vi "amp e offset control.vi"(8 "amp ref":refnum<vi>, 9 "Amplitude (Vp)":dbl, 10 "Offset (V)":dbl, 11 "offset ref":refnum<vi>) -> (1 "Nova Amplitude":dbl, 2 "Novo Offset":dbl)   [LabVIEW 2019]
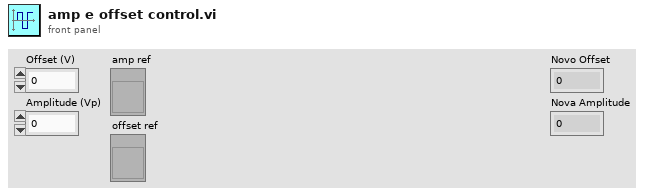
[diagram p1: front panel]
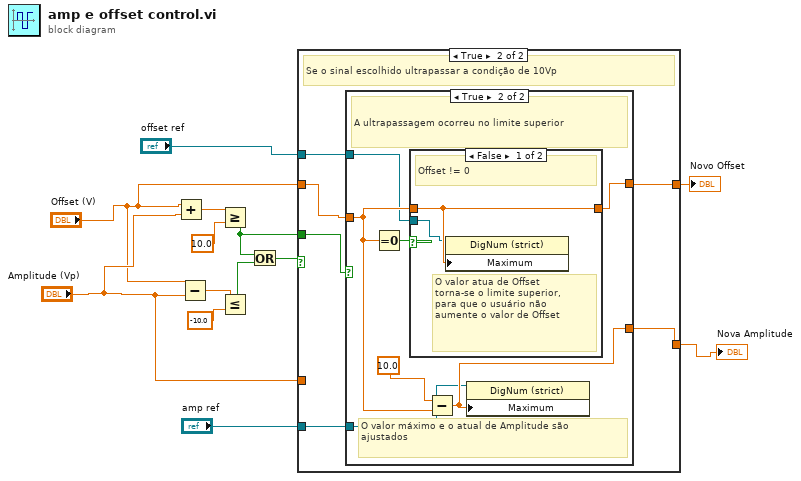
[diagram p0: block diagram]
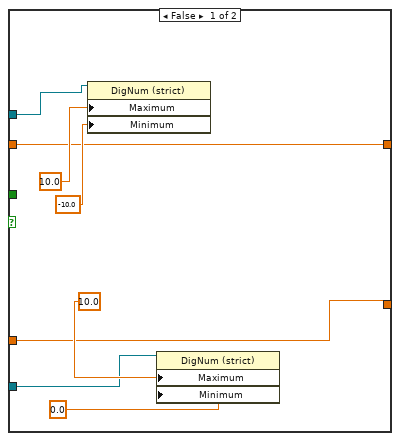
[diagram p2: hidden frame]
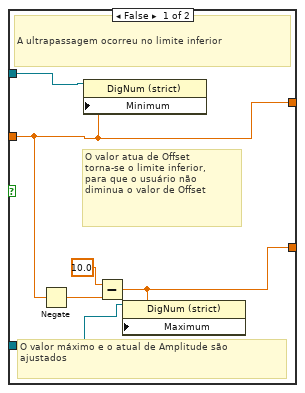
[diagram p3: hidden frame]
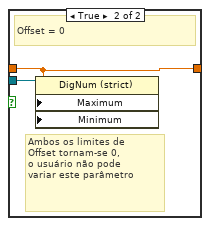
[diagram p4: hidden frame]
diagram:
  n1 = Add(x="Offset (V)", y="Amplitude (Vp)") -> (x+y=w13:dbl)
  n2 = Subtract(x="Offset (V)", y="Amplitude (Vp)") -> (x-y=w11:dbl)
  n3 = Greater Or Equal?(x=w13, y=10.0) -> (x >= y?=w10:bool)
  n4 = Less Or Equal?(x=w11, y=-10.0) -> (x <= y?=w12:bool)
  n5 = Or(x=w10, y=w12) -> (x .or. y?=w9:bool)
  n6 = case shown="True" w9 {
    tunnel: [w17 w26] -> w3
    tunnel: w10 -> [_ w27]
    tunnel: "Offset (V)" -> [w16 w25]
    tunnel: "Amplitude (Vp)" -> [w17 _]
    tunnel: [w16 w24] -> w4
    tunnel: "offset ref" -> [w15 w23]
    tunnel: "amp ref" -> [w14 w22]
    frame False {
      n7 = property on="Property Node" class="DigNum (strict)"(reference=w15, "Maximum"=10.0 ("Data Entry Limits:Maximum"), "Minimum"=-10.0 ("Data Entry Limits:Minimum")) -> ()  [unwired: 1 in, 2 out]
      n8 = property on="Property Node" class="DigNum (strict)"(reference=w14, "Maximum"=10.0 ("Data Entry Limits:Maximum"), "Minimum"=0.0 ("Data Entry Limits:Minimum")) -> ()  [unwired: 1 in, 2 out]
    }
    frame True {
      # "Se o sinal escolhido ultrapassar a condição de 10Vp"
      n9 = case shown="True" w27 {
        tunnel: [w31 w39] -> w26
        tunnel: w25 -> [w30 w37]
        tunnel: [w30 w36] -> w24
        tunnel: w23 -> [w29 w35]
        tunnel: w22 -> [w28 w34]
        frame False {
          # "O valor máximo e o atual de Amplitude são\najustados"
          # "O valor atua de Offset\ntorna-se o limite inferior,\npara que o usuário não \ndiminua o valor de Offset"
          # "A ultrapassagem ocorreu no limite inferior"
          n10 = Negate(x=w30) -> (-x=w32:dbl)
          n11 = property on="Property Node" class="DigNum (strict)"(reference=w29, "Minimum"=w30) -> ()  [unwired: 1 in, 2 out]
          n12 = Subtract(x=10.0, y=w32) -> (x-y=w31:dbl)
          n13 = property on="Property Node" class="DigNum (strict)"(reference=w28, "Maximum"=w31) -> ()  [unwired: 1 in, 2 out]
        }
        frame True {
          # "O valor máximo e o atual de Amplitude são\najustados"
          # "A ultrapassagem ocorreu no limite superior"
          n14 = Equal To 0?(x=w37) -> (x = 0?=w38:bool)
          n15 = case shown="False" w38 {
            tunnel: w37 -> [w42 w44]
            tunnel: [w42 w44] -> w36
            tunnel: w35 -> [w41 w43]
            frame False {
              # "O valor atua de Offset\ntorna-se o limite superior,\npara que o usuário não \naumente o valor de Offset"
              # "Offset != 0"
              n16 = property on="Property Node" class="DigNum (strict)"(reference=w41, "Maximum"=w42) -> ()  [unwired: 1 in, 2 out]
            }
            frame True {
              # "Ambos os limites de\nOffset tornam-se 0,\no usuário não pode\nvariar este parâmetro"
              # "Offset = 0"
              n17 = property on="Property Node" class="DigNum (strict)"(reference=w43, "Maximum"=w44, "Minimum"=w44) -> ()  [unwired: 1 in, 2 out]
            }
          }
          n18 = Subtract(x=10.0, y=w37) -> (x-y=w39:dbl)
          n19 = property on="Property Node" class="DigNum (strict)"(reference=w34, "Maximum"=w39) -> ()  [unwired: 1 in, 2 out]
        }
      }
    }
  }
  "Novo Offset" <- w4
  "Nova Amplitude" <- w3
